vi "myRIO__TCP_constants_byteRange_messageType.vi"() -> (6 "output_Start_char":string="S", 8 "output_Start_byte":u8=83, 10 "output_Quit_char":string="Q", 11 "output_analogInput_char":string="I", 12 "output_Quit_byte":u8=81, 13 "output_analogInput_byte":u8=73, 14 "output_Block_char":string="B", 15 "output_Block_byte":u8=66, 16 "output_Trial_char":string="T", 17 "output_Trial_byte":u8=84, 18 "output_selectResponse_char":string="R", 19 "output_selectResponse_byte":u8=82)   [LabVIEW 2014]
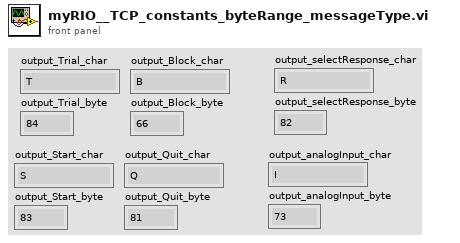
[diagram p1: front panel]
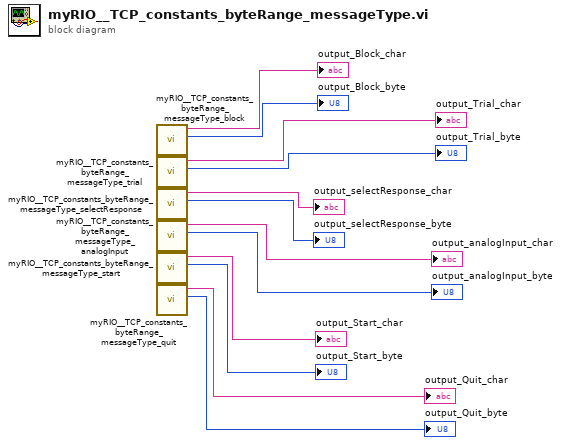
[diagram p0: block diagram]
diagram:
  n1 = call "myRIO__TCP_constants_byteRange_messageType_block.vi"() -> ("output_Block_byte"=→"output_Block_byte":u8, "output_Block_char"=→"output_Block_char":string)  [unwired: 10 in]
  n2 = call "myRIO__TCP_constants_byteRange_messageType_trial.vi"() -> ("output_Trial_byte"=→"output_Trial_byte":u8, "output_Trial_char"=→"output_Trial_char":string)  [unwired: 10 in]
  n3 = call "myRIO__TCP_constants_byteRange_messageType_selectResponse.vi"() -> ("output_selResponse_byte"=→"output_selectResponse_byte":u8, "output_selectResponse_char"=→"output_selectResponse_char":string)  [unwired: 10 in]
  n4 = call "myRIO__TCP_constants_byteRange_messageType_analogInput.vi"() -> ("output_analogInput_byte"=→"output_analogInput_byte":u8, "output_analogInput_char"=→"output_analogInput_char":string)  [unwired: 10 in]
  n5 = call "myRIO__TCP_constants_byteRange_messageType_start.vi"() -> ("output_Start_byte"=→"output_Start_byte":u8, "output_Start_char"=→"output_Start_char":string)  [unwired: 10 in]
  n6 = call "myRIO__TCP_constants_byteRange_messageType_quit.vi"() -> ("output_Quit_byte"=→"output_Quit_byte":u8, "output_Quit_char"=→"output_Quit_char":string)  [unwired: 10 in]
